vi "Read As Stream_Sync.vi"(7 "CloseDestinationStream [T]":bool=TRUE, 8 "error in (no error)":errorcluster, 10 "stream":refnum<k24>, 11 "HttpContent in":refnum<class "HttpContent.lvclass">) -> (0 "error out":errorcluster, 1 "IsCompleted":bool, 3 "HttpContent out":refnum<class "HttpContent.lvclass">, 4 "Canceled":bool)   [LabVIEW 2018, in "HttpClient_NET.lvlib" / "HttpContent.lvclass"]
doc: "<b> </b> <b> </b>\nHttpClient_NET\nJustin Young - Viviota\nCopyright (c) 2021\nLicense: BSD"
uses:
  HttpContent.lvclass
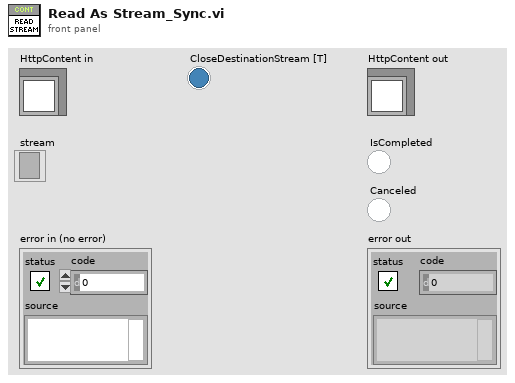
[diagram p1: front panel]
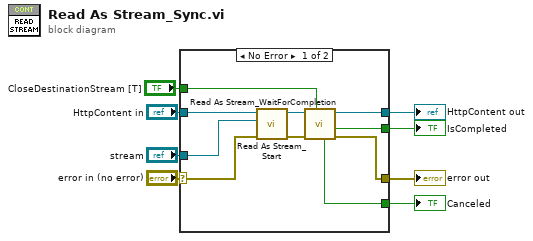
[diagram p0: block diagram]
diagram:
  n1 = case shown="No Error" "error in (no error)" {
    selector: "error in (no error)" -> [w16 w20]
    tunnel: [w15 w20] -> w7
    tunnel: [w12 w19] -> w5
    tunnel: "HttpContent in" -> [w18 w19]
    tunnel: "stream" -> [w14 _]
    tunnel: [w11 _] -> w3
    tunnel: [w10 _] -> w2
    tunnel: "CloseDestinationStream [T]" -> [w9 _]
    frame No Error {
      n2 = call "Read As Stream_Start.vi"("error in (no error)"=w16, "DestinationStream"=w14, "HttpContent in"=w18) -> ("error out"=w13:errorcluster, "HttpContent out"=w17:refnum<class "HttpContent.lvclass">)  [unwired: 7 in]
      n3 = call "Read As Stream_WaitForCompletion.vi"("CloseDestinationStream [T]"=w9, "error in (no error)"=w13, "HttpContent in"=w17) -> ("error out"=w15:errorcluster, "IsCompleted"=w10:bool, "HttpContent out"=w12:refnum<class "HttpContent.lvclass">, "Canceled"=w11:bool)  [unwired: 5 in]
    }
    frame Error {
    }
  }
  "error out" <- w7
  "HttpContent out" <- w5
  "IsCompleted" <- w2
  "Canceled" <- w3
